vi "SVG2emf-command.vi"(8 "Error in":errorcluster caption="Error in (no error)", 10 "EMF路径":path, 11 "SVG路径":path) -> (0 "Error out":errorcluster)   [LabVIEW 2017]
uses:
  Microsoft.Office.Interop.Visio
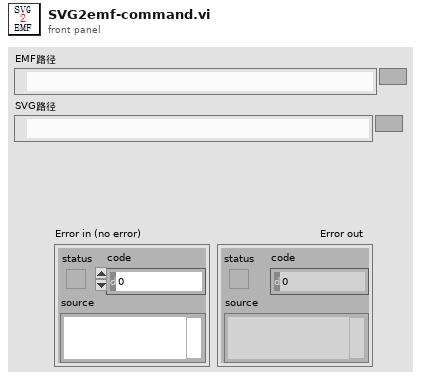
[diagram p1: front panel]
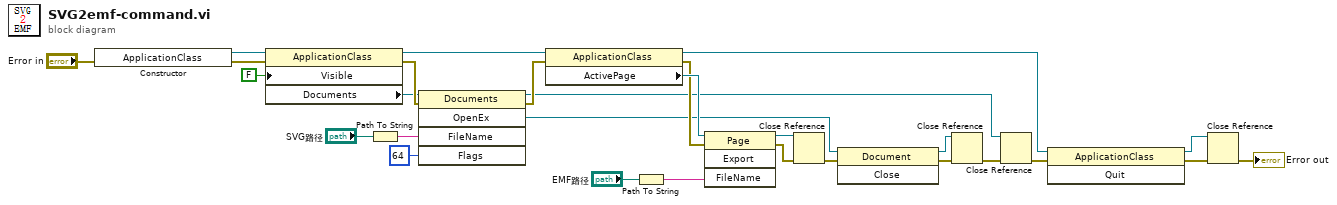
[diagram p0: block diagram]
diagram:
  n1 = constructor class="ApplicationClass"(error in="Error in") -> (reference out=w27:refnum<k24>, error out=w28:errorcluster)  [unwired: 2 in, 1 out]
  n2 = property on="属性节点" class="ApplicationClass"(reference=w27, error in=w28, "Visible"=FALSE) -> (reference out=w14:refnum<k24>, error out=w26:errorcluster, "Documents"=w20:refnum<k24>)
  n3 = Path To String(path="SVG路径") -> (string=w25:string)
  n4 = invoke class="Documents" method="OpenEx"(reference=w20, error in=w26, "FileName"=w25, "Flags"=i16 64) -> (reference out=w12:refnum<k24>, error out=w16:errorcluster, "OpenEx"=w5:refnum<k24>)  [unwired: 1 in, 2 out]
  n5 = property class="ApplicationClass"(reference=w14, error in=w16) -> (reference out=w7:refnum<k24>, error out=w13:errorcluster, "ActivePage"=w15:refnum<k24>)
  n6 = Path To String(path="EMF路径") -> (string=w22:string)
  n7 = invoke class="Page" method="Export"(reference=w15, error in=w13, "FileName"=w22) -> (reference out=w11:refnum<k24>, error out=w10:errorcluster)  [unwired: 1 in, 2 out]
  n8 = Close Reference(reference=w11, error in (no error)=w10) -> (error out=w8:errorcluster)
  n9 = invoke class="Document" method="Close"(reference=w5, error in=w8) -> (reference out=w3:refnum<k24>, error out=w6:errorcluster)  [unwired: 1 in, 1 out]
  n10 = Close Reference(reference=w3, error in (no error)=w6) -> (error out=w4:errorcluster)
  n11 = Close Reference(reference=w12, error in (no error)=w4) -> (error out=w9:errorcluster)
  n12 = invoke on="调用节点" class="ApplicationClass" method="Quit"(reference=w7, error in=w9) -> (reference out=w18:refnum<k24>, error out=w17:errorcluster)  [unwired: 1 in, 1 out]
  n13 = Close Reference(reference=w18, error in (no error)=w17) -> (error out=→"Error out":errorcluster)
